vi "PTScanner.new alg.vi"() -> ()   [LabVIEW 2012, in "PTScanner.lvlib"]
uses:
  PTScanner.lvlib
  PTScanner.step obj parameters.ctl
panel:
  out "Steps out 2":T2(array[cluster])
  out "Array":i32[](array[numeric])
  in  "Steps":T2(array[cluster])
  out "Steps out":T2(array[cluster])
  in  "Object table":dbl[][](array[numeric])
  in  "Sizes":i32[](array[numeric])
  in  "Step":cluster{"Finished":bool, "object's setup":T1[]}
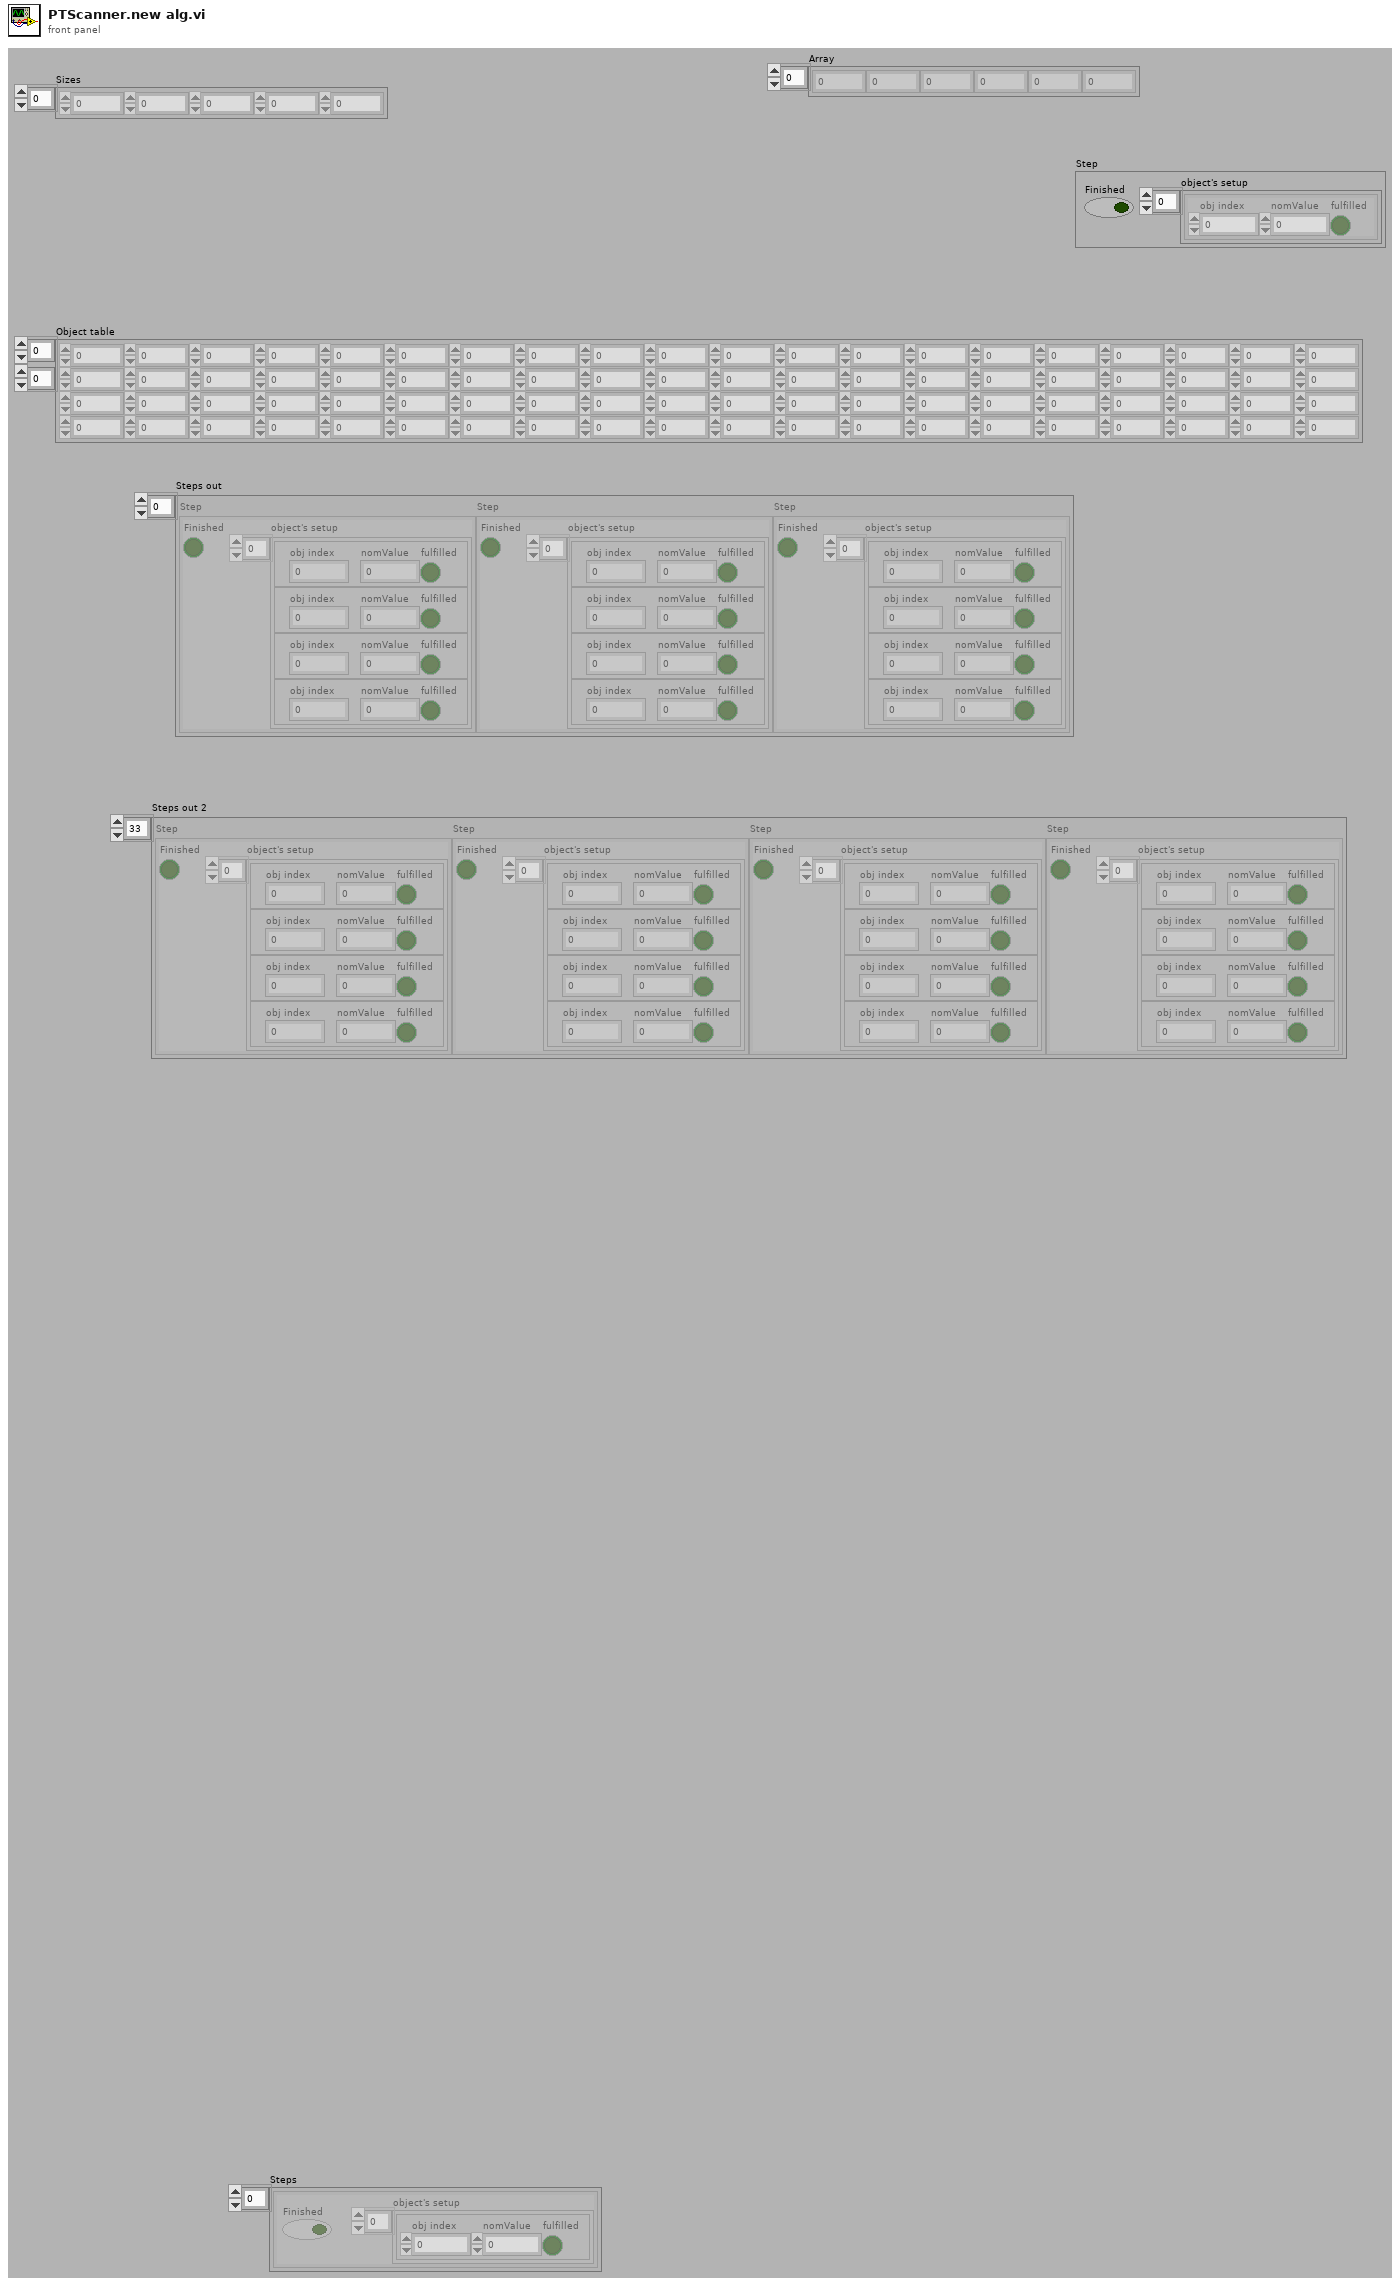
[diagram p1: front panel]
types:
  T1 = typedef "PTScanner.lvlib/PTScanner.step obj parameters.ctl" = cluster{"obj index":i32, "nomValue":dbl, "fulfilled":bool}
  T2 = cluster{"Finished":bool, "object's setup":T1[]}[]
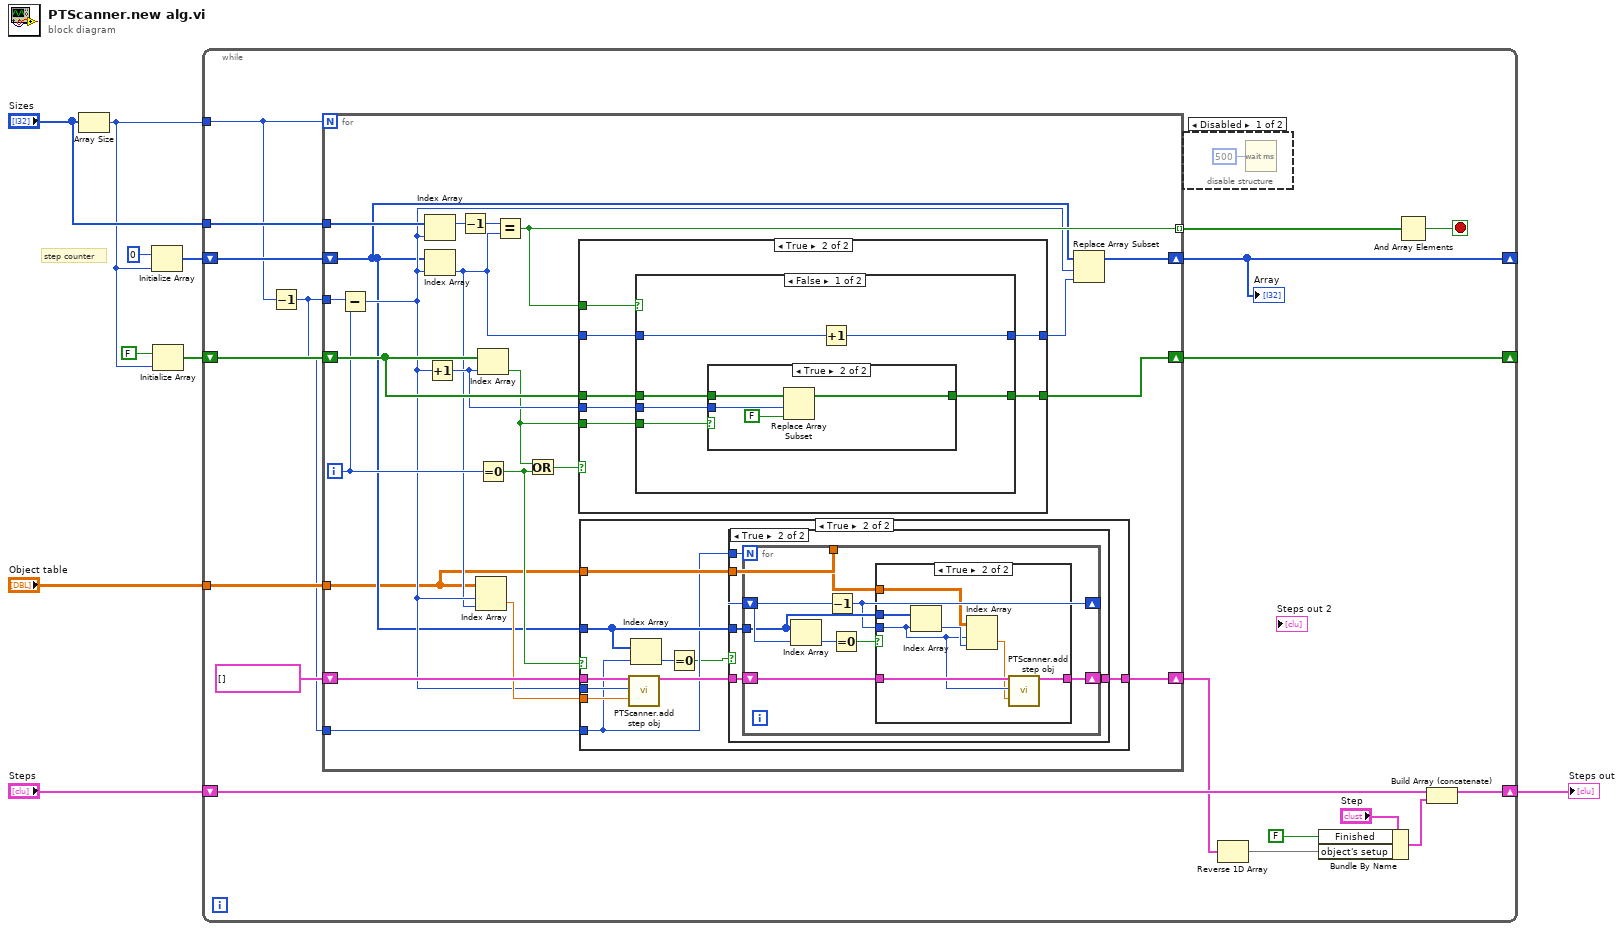
[diagram p0: block diagram]
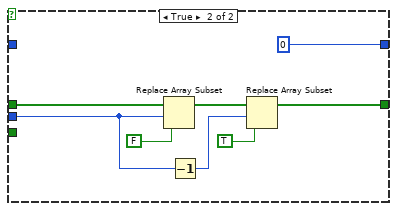
[diagram p8: hidden frame]
diagram:
  # "step counter"
  n1 = Array Size(array="Sizes") -> (size(s)=w1:i32)
  n2 = Initialize Array(0, w1) -> (w6:i32[])
  n3 = Initialize Array(FALSE, w1) -> (w5:bool[])
  n4 = while {
    tunnel: "Sizes" -> [w22]
    shift-right: [w10] -> _
    shift-left: w6 -> [w25]
    tunnel: "Object table" -> [w24]
    shift-right: [w20] -> w2
    shift-left: "Steps" -> [w23]
    shift-right: [w18] -> _
    shift-left: w5 -> [w21]
    tunnel: w1 -> [w19]
    stop <- w26 stop-if-true
    n5 = Decrement(x=w19) -> (x-1=w11:i32)
    n6 = for {
      N: w19 -> [_]
      tunnel: w22 -> [w49]
      tunnel: [w41] -> w27 mode=indexing
      tunnel: w24 -> [w30]
      tunnel: w11 -> [w48]
      shift-right: [w34] -> w10
      shift-left: w25 -> [w31]
      shift-right: [w42] -> w18
      shift-left: w21 -> [w44]
      shift-right: [w32] -> w16
      shift-left: T1[] [] ("Array") -> [w38]
      tunnel: w11 -> [w29]
      i -> [w39]
      n7 = Subtract(x=w48, y=w39) -> (x-y=w35:i32)
      n8 = Index Array(array=w49, index=w35) -> (element=w47:i32)
      n9 = Index Array(array=w31, index=w35) -> (element=w33:i32)
      n10 = Increment(x=w35) -> (x+1=w43:i32)
      n11 = Decrement(x=w47) -> (x-1=w50:i32)
      n12 = Index Array(array=w30, index (row)=w35, index (col)=w33) -> (element=w37:dbl)
      n13 = Index Array(array=w44, index=w43) -> (element=w40:bool)
      n14 = Equal To 0?(x=w39) -> (x = 0?=w36:bool)
      n15 = Equal?(x=w50, y=w33) -> (x = y?=w41:bool)
      n16 = Or(x=w40, y=w36) -> (x .or. y?=w46:bool)
      n17 = case shown="True" w46 {
        tunnel: w33 -> [w85 w86]
        tunnel: [w85 w92] -> w45
        tunnel: w44 -> [w84 w91]
        tunnel: w43 -> [_ w90]
        tunnel: [w84 w89] -> w42
        tunnel: w40 -> [_ w88]
        tunnel: w41 -> [_ w87]
        frame False {
        }
        frame True {
          n18 = case shown="False" w87 {
            tunnel: w86 -> [w98 _]
            tunnel: [w97 0] -> w92
            tunnel: w91 -> [w96 w109]
            tunnel: w90 -> [w94 w106]
            tunnel: [w95 w105] -> w89
            tunnel: w88 -> [w93 _]
            frame False {
              n19 = case shown="True" w93 {
                tunnel: w96 -> [w99 w103]
                tunnel: w94 -> [_ w100]
                tunnel: [w99 w102] -> w95
                frame False {
                }
                frame True {
                  n20 = Replace Array Subset(array=w103, new element=FALSE, index=w100) -> (w102:bool[])
                }
              }
              n21 = Increment(x=w98) -> (x+1=w97:i32)
            }
            frame True {
              n22 = Replace Array Subset(array=w109, new element=FALSE, index=w106) -> (w110:bool[])
              n23 = Decrement(x=w106) -> (x-1=w104:i32)
              n24 = Replace Array Subset(array=w110, new element=TRUE, index=w104) -> (w105:bool[])
            }
          }
        }
      }
      n25 = case shown="True" w36 {
        tunnel: w38 -> [w51 w61]
        tunnel: [w51 w57] -> w32
        tunnel: w35 -> [_ w60]
        tunnel: w37 -> [_ w59]
        tunnel: w31 -> [_ w55]
        tunnel: w30 -> [_ w56]
        tunnel: w29 -> [_ w54]
        frame False {
        }
        frame True {
          n26 = call "PTScanner.add step obj.vi"("array"=w61, "obj index"=w60, "nomValue"=w59) -> ("appended array"=w58:T1[])  [unwired: 16 in]
          n27 = Index Array(array=w55, index=w54) -> (element=w53:i32)
          n28 = Equal To 0?(x=w53) -> (x = 0?=w52:bool)
          n29 = case shown="True" w52 {
            tunnel: w58 -> [w62 w67]
            tunnel: [w62 w66] -> w57
            tunnel: w56 -> [_ w65]
            tunnel: w55 -> [_ w64]
            tunnel: w54 -> [_ w63]
            frame False {
            }
            frame True {
              n30 = for {
                N: w63 -> [_]
                tunnel: w64 -> [w70]
                shift-right: [w69] -> _
                shift-left: w63 -> [w75]
                shift-right: [w71] -> w66
                shift-left: w67 -> [w72]
                tunnel: w65 -> [w68]
                n31 = Index Array(array=w70, index=w75) -> (element=w74:i32)
                n32 = Decrement(x=w75) -> (x-1=w69:i32)
                n33 = Equal To 0?(x=w74) -> (x = 0?=w73:bool)
                n34 = case shown="True" w73 {
                  tunnel: w72 -> [w76 w80]
                  tunnel: [w76 w79] -> w71
                  tunnel: w70 -> [_ w83]
                  tunnel: w69 -> [_ w78]
                  tunnel: w68 -> [_ w81]
                  frame False {
                  }
                  frame True {
                    n35 = Index Array(array=w83, index=w78) -> (element=w82:i32)
                    n36 = Index Array(array=w81, index (row)=w78, index (col)=w82) -> (element=w77:dbl)
                    n37 = call "PTScanner.add step obj.vi"("array"=w80, "obj index"=w78, "nomValue"=w77) -> ("appended array"=w79:T1[])  [unwired: 16 in]
                  }
                }
              }
            }
          }
        }
      }
      n38 = Replace Array Subset(array=w31, new element=w45, index=w35) -> (w34:i32[])
    }
    "Array" <- w10
    n39 = disable-structure shown="Disabled" {
      frame Disabled {
        n40 = Wait (ms)(milliseconds to wait=u32 500) -> ()  [unwired: 1 out]
      }
      frame Enabled {
      }
    }
    n41 = Reverse 1D Array(array=w16) -> (reversed array=w12:T1[])
    n42 = Bundle By Name(cluster="Step", "Finished"=FALSE, "object's setup"=w12) -> (w13:cluster{"Finished":bool, "object's setup":T1[]})
    n43 = And Array Elements(Boolean array=w27) -> (logical AND=w26:bool)
    n44 = Build Array (concatenate)(w23, w13) -> (w20:T2)
  }
  "Steps out" <- w2
